vi "Close GUI.vi"(8 "Error In":errorcluster, 10 "Close GUI Option (Default = \"In dev env, don't close if top-level caller\")":T1=enum."In dev env, don't close if top-level caller", 11 "VI Refnum":refnum<vi>) -> (0 "Error Out":errorcluster)   [LabVIEW 2023, in "Error Manager.lvlib"]
doc: "This VI closes the Front Panel (the GUI) of the VI whose refnum is passed as an argument to the \"VI Refnum\" input (usually, the immediate caller VI).\n\nError behaviour: This VI executes even if an error is passed as an argument to the \"Error In\" terminal."
uses:
  Error Manager.lvlib
  Close GUI Option (Enum).ctl
panel:
  out "Top-Level Caller Qualified Name":string
  out "Call Chain":string[](array[string])
  # "Development\ncontrols/indicators useful for development and testing, but which are not outputs of the VI"
  # "Input\nInputs to the VI"
  # "Output\nOutputs of the VI"
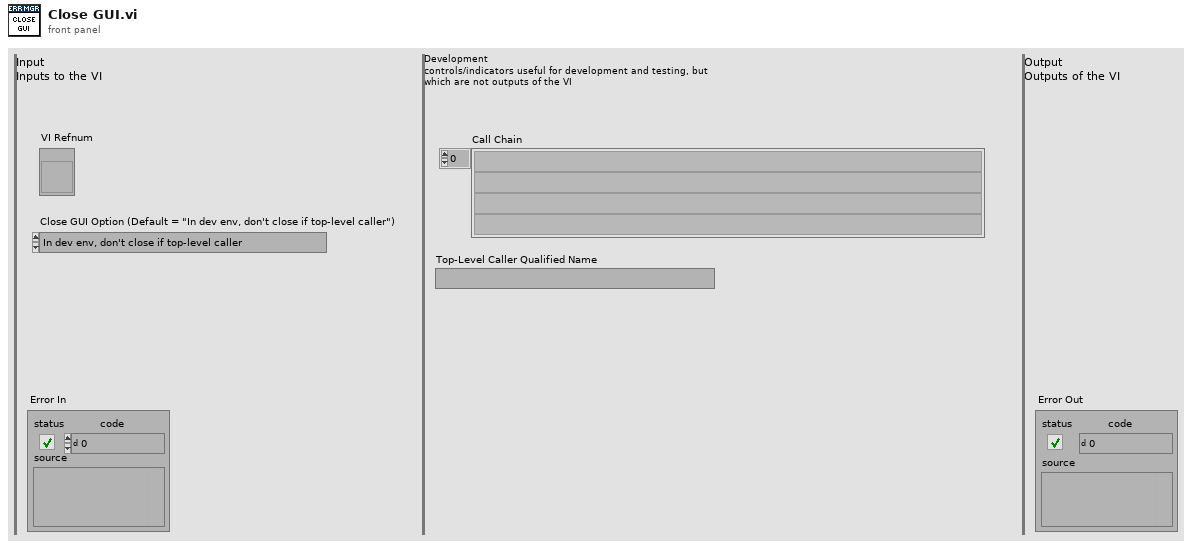
[diagram p1: front panel]
types:
  T1 = typedef "Error Manager.lvlib/Close GUI Option (Enum).ctl" = enum16{"In dev env, don't close", "In dev env, don't close if top-level caller", "Close Always"}
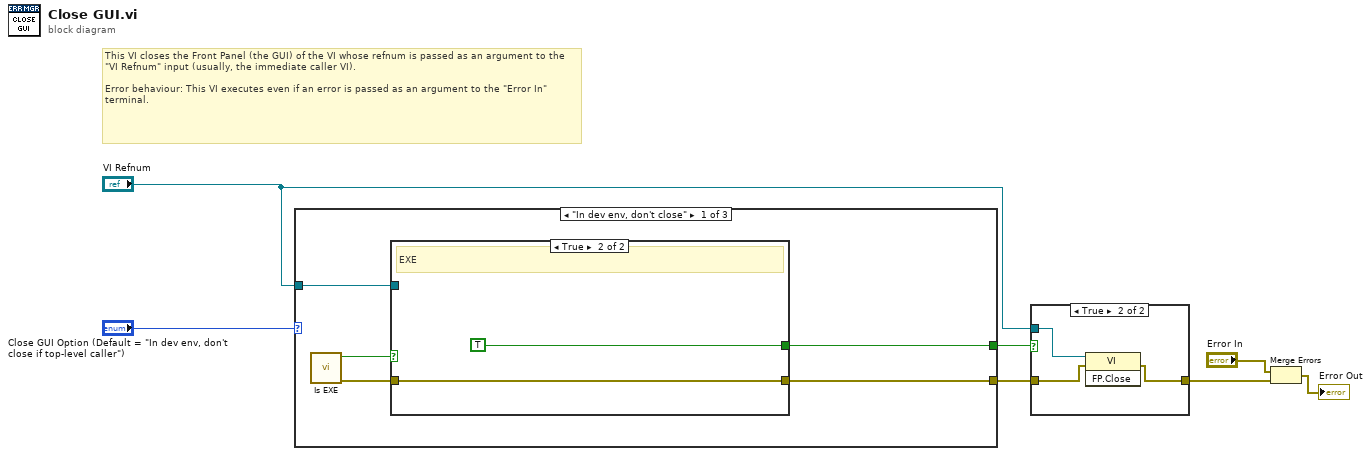
[diagram p0: block diagram]
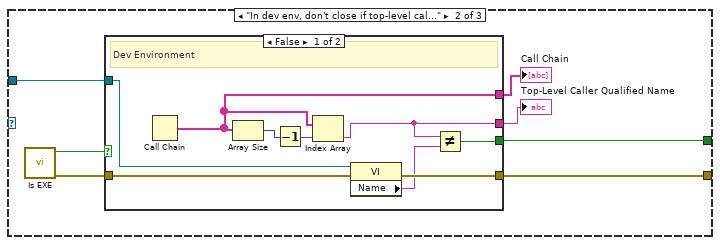
[diagram p3: hidden frame]
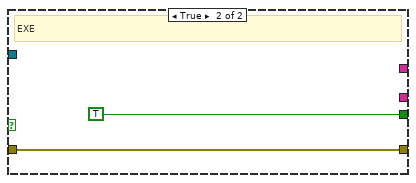
[diagram p4: hidden frame]
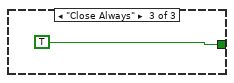
[diagram p5: hidden frame]
diagram:
  # "This VI closes the Front Panel (the GUI) of the VI whose refnum is passed as an argument to the \"VI Refnum\" input (usually, the immediate caller VI).\n\nError behaviour: This VI executes even if an error is passed as an argument to the \"Error In\" terminal."
  n1 = case shown="\"In dev env, don't close\"" "Close GUI Option (Default = \"In dev env, don't close if top-level caller\")" {
    tunnel: [w11 w21 _] -> w4
    tunnel: [w9 w19 TRUE] -> w3
    tunnel: "VI Refnum" -> [w8 w18 _]
    frame "In dev env, don't close" {
      n2 = call "Is EXE.vi"() -> ("error out"=w12:errorcluster, "T = is EXE"=w10:bool)  [unwired: 9 in, 1 out]
      n3 = case shown="True" w10 {
        tunnel: w12 -> [w13 w15]
        tunnel: [w13 w15] -> w11
        tunnel: [_ TRUE] -> w9
        tunnel: w8 -> [_ _]
        frame False {
          # "Dev Environment"
        }
        frame True {
          # "EXE"
        }
      }
    }
    frame "In dev env, don't close if top-level caller" {
      n4 = call "Is EXE.vi"() -> ("error out"=w22:errorcluster, "T = is EXE"=w20:bool)  [unwired: 9 in, 1 out]
      n5 = case shown="False" w20 {
        tunnel: w22 -> [w31 w33]
        tunnel: [w27 w33] -> w21
        tunnel: [w23 TRUE] -> w19
        tunnel: [w29 _] -> w17
        tunnel: w18 -> [w26 _]
        tunnel: [w25 _] -> w16
        frame False {
          # "Dev Environment"
          n6 = Call Chain() -> (call chain=w29:string[])
          n7 = Array Size(array=w29) -> (size(s)=w30:i32)
          n8 = Decrement(x=w30) -> (x-1=w28:i32)
          n9 = Index Array(array=w29, index=w28) -> (element=w25:string)
          n10 = property class="VI"(reference=w26, error in=w31) -> (error out=w27:errorcluster, "Name"=w24:string)  [unwired: 1 out]
          n11 = Not Equal?(x=w25, y=w24) -> (x != y?=w23:bool)
        }
        frame True {
          # "EXE"
        }
      }
      "Call Chain" <- w17
      "Top-Level Caller Qualified Name" <- w16
    }
    frame "Close Always" {
    }
  }
  n12 = case shown="True" w3 {
    tunnel: [w35 w38] -> w7
    tunnel: "VI Refnum" -> [_ w37]
    tunnel: w4 -> [w35 w36]
    frame False {
    }
    frame True {
      n13 = invoke class="VI" method="FP.Close"(reference=w37, error in=w36) -> (error out=w38:errorcluster)  [unwired: 1 in, 2 out]
    }
  }
  n14 = Merge Errors("Error In", w7) -> (→"Error Out":errorcluster)
